vi "Initialise.vi"(8 "error in (no error)":errorcluster, 11 "Instrument in":refnum<class "Instrument.lvclass">) -> (0 "error out":errorcluster, 2 "Status":string, 3 "Instrument out":refnum<class "Instrument.lvclass">)   [LabVIEW 2020, in "Instrument.lvclass"]
uses:
  Instrument.lvclass
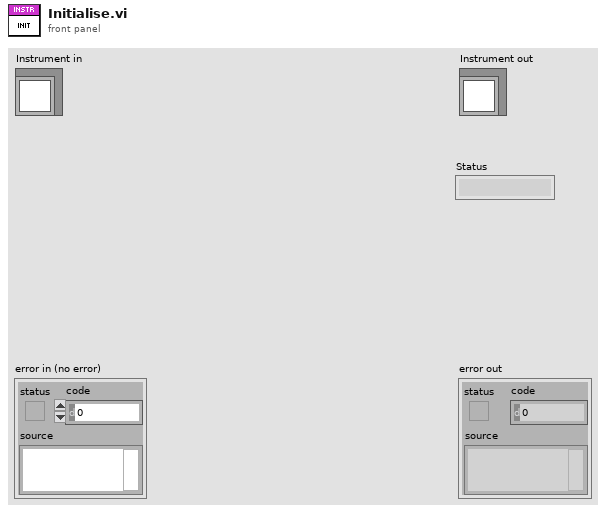
[diagram p1: front panel]
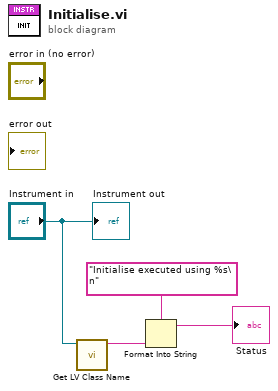
[diagram p0: block diagram]
diagram:
  n1 = call <vilib>:"Get LV Class Name.vi"("object"="Instrument in") -> ("class name"=w2:string)  [unwired: 9 in, 1 out]
  n2 = Format Into String(format string="Initialise executed using %s\n", w2) -> (resulting string=→"Status":string)  [unwired: 2 in, 1 out]
  "Instrument out" <- "Instrument in"
